vi "Wait On Lock.vi"(7 "Lock Type":T1, 8 "error in (no error)":errorcluster, 9 "Timeout ms":i32, 11 "WebsocketStream in":refnum<class "WebsocketStream.lvclass">) -> (0 "error out":errorcluster, 1 "Remaining  Timeout":i32, 2 "Timeout":bool, 3 "WebsocketStream out":refnum<class "WebsocketStream.lvclass">)   [LabVIEW 2020, in "Stream-Websocket.lvlib" / "WebsocketStream.lvclass"]
uses:
  WebsocketStream.lvclass
  Lock Type.ctl
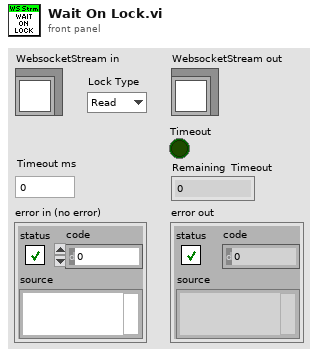
[diagram p1: front panel]
types:
  T1 = typedef "Stream-Websocket.lvlib/WebsocketStream.lvclass/Lock Type.ctl" = enum16{"Read", "Write"}
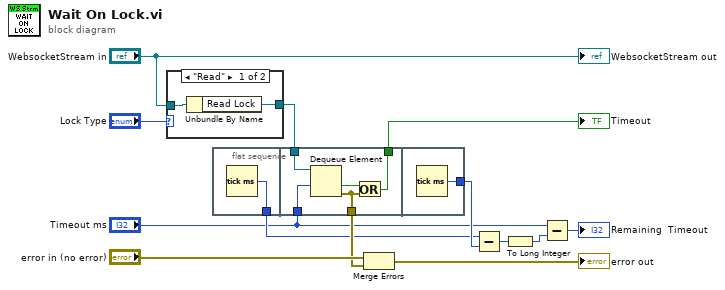
[diagram p0: block diagram]
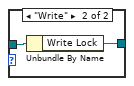
[diagram p2: hidden frame]
diagram:
  n1 = case shown="\"Read\"" "Lock Type" {
    tunnel: "WebsocketStream in" -> [w15 w17]
    tunnel: [w14 w16] -> w12
    frame "Read" {
      n2 = Unbundle By Name(w15) -> ("Read Lock"=w14:refnum<queue>)
    }
    frame "Write" {
      n3 = Unbundle By Name(w17) -> ("Write Lock"=w16:refnum<queue>)
    }
  }
  n4 = flat-sequence {
    tunnel: [w18] -> w6
    tunnel: w12 -> [w23]
    tunnel: [w20] -> w10
    tunnel: [w19] -> w9
    tunnel: "Timeout ms" -> [w22]
    tunnel: [w24] -> w7
    frame #0 {
      n5 = Tick Count (ms)() -> (millisecond timer value=w18:u32)
    }
    frame #1 {
      n6 = Dequeue Element(queue=w23, timeout in ms (-1)=w22) -> (timed out?=w21:bool, error out=w20:errorcluster)  [unwired: 1 in, 2 out]
      n7 = Or(x=w21, y=w20) -> (x .or. y?=w19:bool)
    }
    frame #2 {
      n8 = Tick Count (ms)() -> (millisecond timer value=w24:u32)
    }
  }
  n9 = Merge Errors("error in (no error)", w10) -> (→"error out":errorcluster)
  n10 = Subtract(x=w6, y=w7) -> (x-y=w4:u32)
  n11 = To Long Integer(number=w4) -> (32bit integer=w3:i32)
  n12 = Subtract(x="Timeout ms", y=w3) -> (x-y=→"Remaining  Timeout":i32)
  "WebsocketStream out" <- "WebsocketStream in"
  "Timeout" <- w9
